vi "P116WriteAuto.vi"(8 "error in (no error)":errorcluster, 9 "NuevoRT":T1, 10 "NuevoSP":T1, 11 "Comunicaciones":T2={"Flujo_1"="ASRL6::INSTR", "Brk1"=FALSE, "Flujo_2"="ASRL6::INSTR", "Brk2"=FALSE, "Flujo_3"="ASRL6::INSTR", "Brk3"=FALSE, "Flujo_4"="ASRL6::INSTR", "Brk4"=FALSE, "Eurothe"="ASRL6::INSTR", "Eurot"=FALSE, "Balanza"="ASRL6::INSTR", "Bal"=FALSE, "eValPos"="ASRL6::INSTR", "eVal"=FALSE, "flowbus"="ASRL6::INSTR", "fb"=FALSE}) -> (0 "error out":errorcluster, 1 "NuevoRT2":T1, 2 "NuevoSP2":T1)   [LabVIEW 2013]
uses:
  4xP116.ctl
  Controles/P2018 Com Control.ctl
  Eurotherm_Hardware_Module Control.ctl
  P2022 TB INCAR GLOBALES.vi
panel:
  out "arrayRT":dbl[](array[numeric])
  out "arraySP":dbl[](array[numeric])
  out "PV":T1
  out "WorkingSP":T1
  out "TargetSP":T1
  in  "Cancel":bool
  in  "Write":bool
  out "Enable(T)":bool=TRUE
  out "VISA Promux":refnum<visa-resource-name>
  in  "Delay Time (s)":dbl=0.1
  # "Programando controladores P116"
  # "C"
  # "ARRIBA"
  # "C/min"
  # "C"
  # "ABAJO"
  # "C/min"
  # "C"
  # "CINTAS"
  # "C/min"
  # "C"
  # "LECTOR"
  # "C/min"
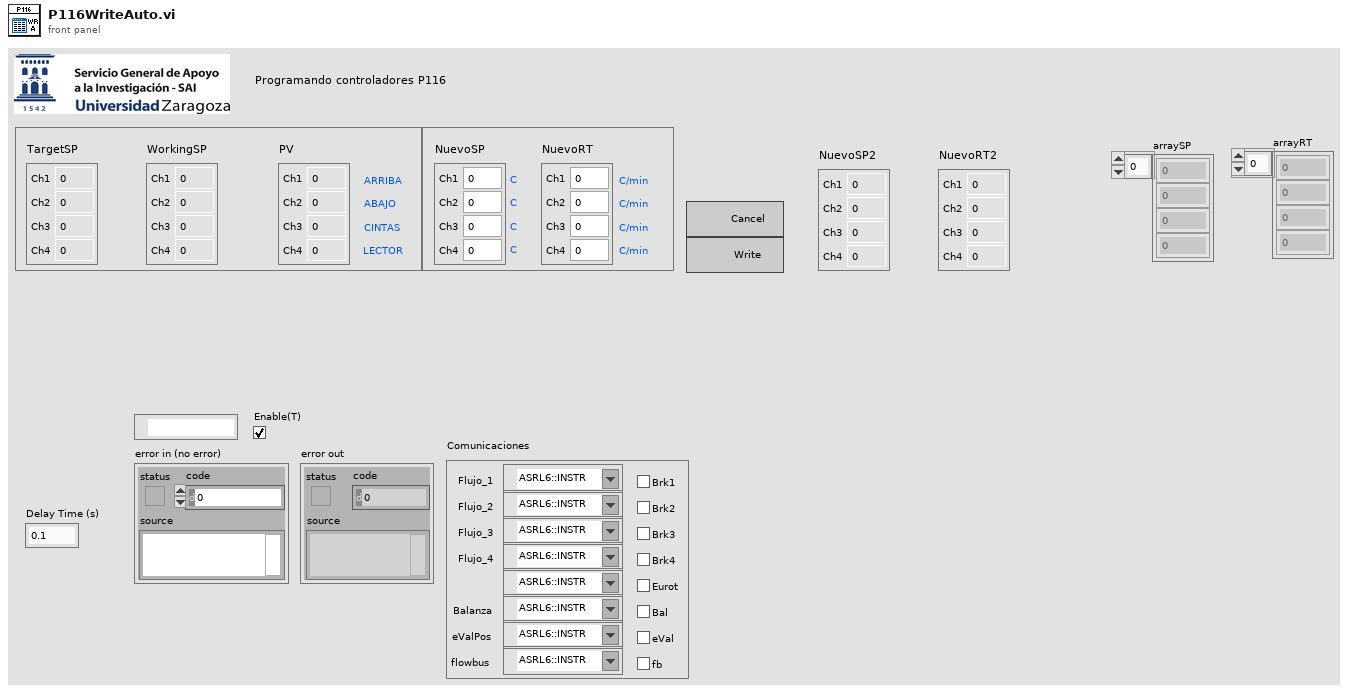
[diagram p1: front panel]
types:
  T1 = typedef "4xP116.ctl" = cluster{"Ch1":dbl, "Ch2":dbl, "Ch3":dbl, "Ch4":dbl}
  T2 = typedef "P2018 Com Control.ctl" = cluster{"Flujo_1":refnum<visa-resource-name>, "Brk1":bool, "Flujo_2":refnum<visa-resource-name>, "Brk2":bool, "Flujo_3":refnum<visa-resource-name>, "Brk3":bool, "Flujo_4":refnum<visa-resource-name>, "Brk4":bool, "Eurothe":refnum<visa-resource-name>, "Eurot":bool, "Balanza":refnum<visa-resource-name>, "Bal":bool, "eValPos":refnum<visa-resource-name>, "eVal":bool, "flowbus":refnum<visa-resource-name>, "fb":bool}
  T3 = typedef "P2018 Eurotherm Control.ctl" = cluster{"TargetSP":T1, "WorkingSP":T1, "Temperatura":T1, "Error":bool, "Date":string, "Delay(s)":dbl, "RateSP":T1, "Potencia":T1}
  T4 = typedef "Eurotherm_Hardware_Module Control.ctl" = enum16{"Initialize", "Write SP", "Read SP+PV", "Write Rate", "Set P", "Set I", "Set D", "Shutdown"}
  T5 = enum16{"Add 1", "Add 2", "Add 10", "Add 11", "Add 12", "Add 13"}[]
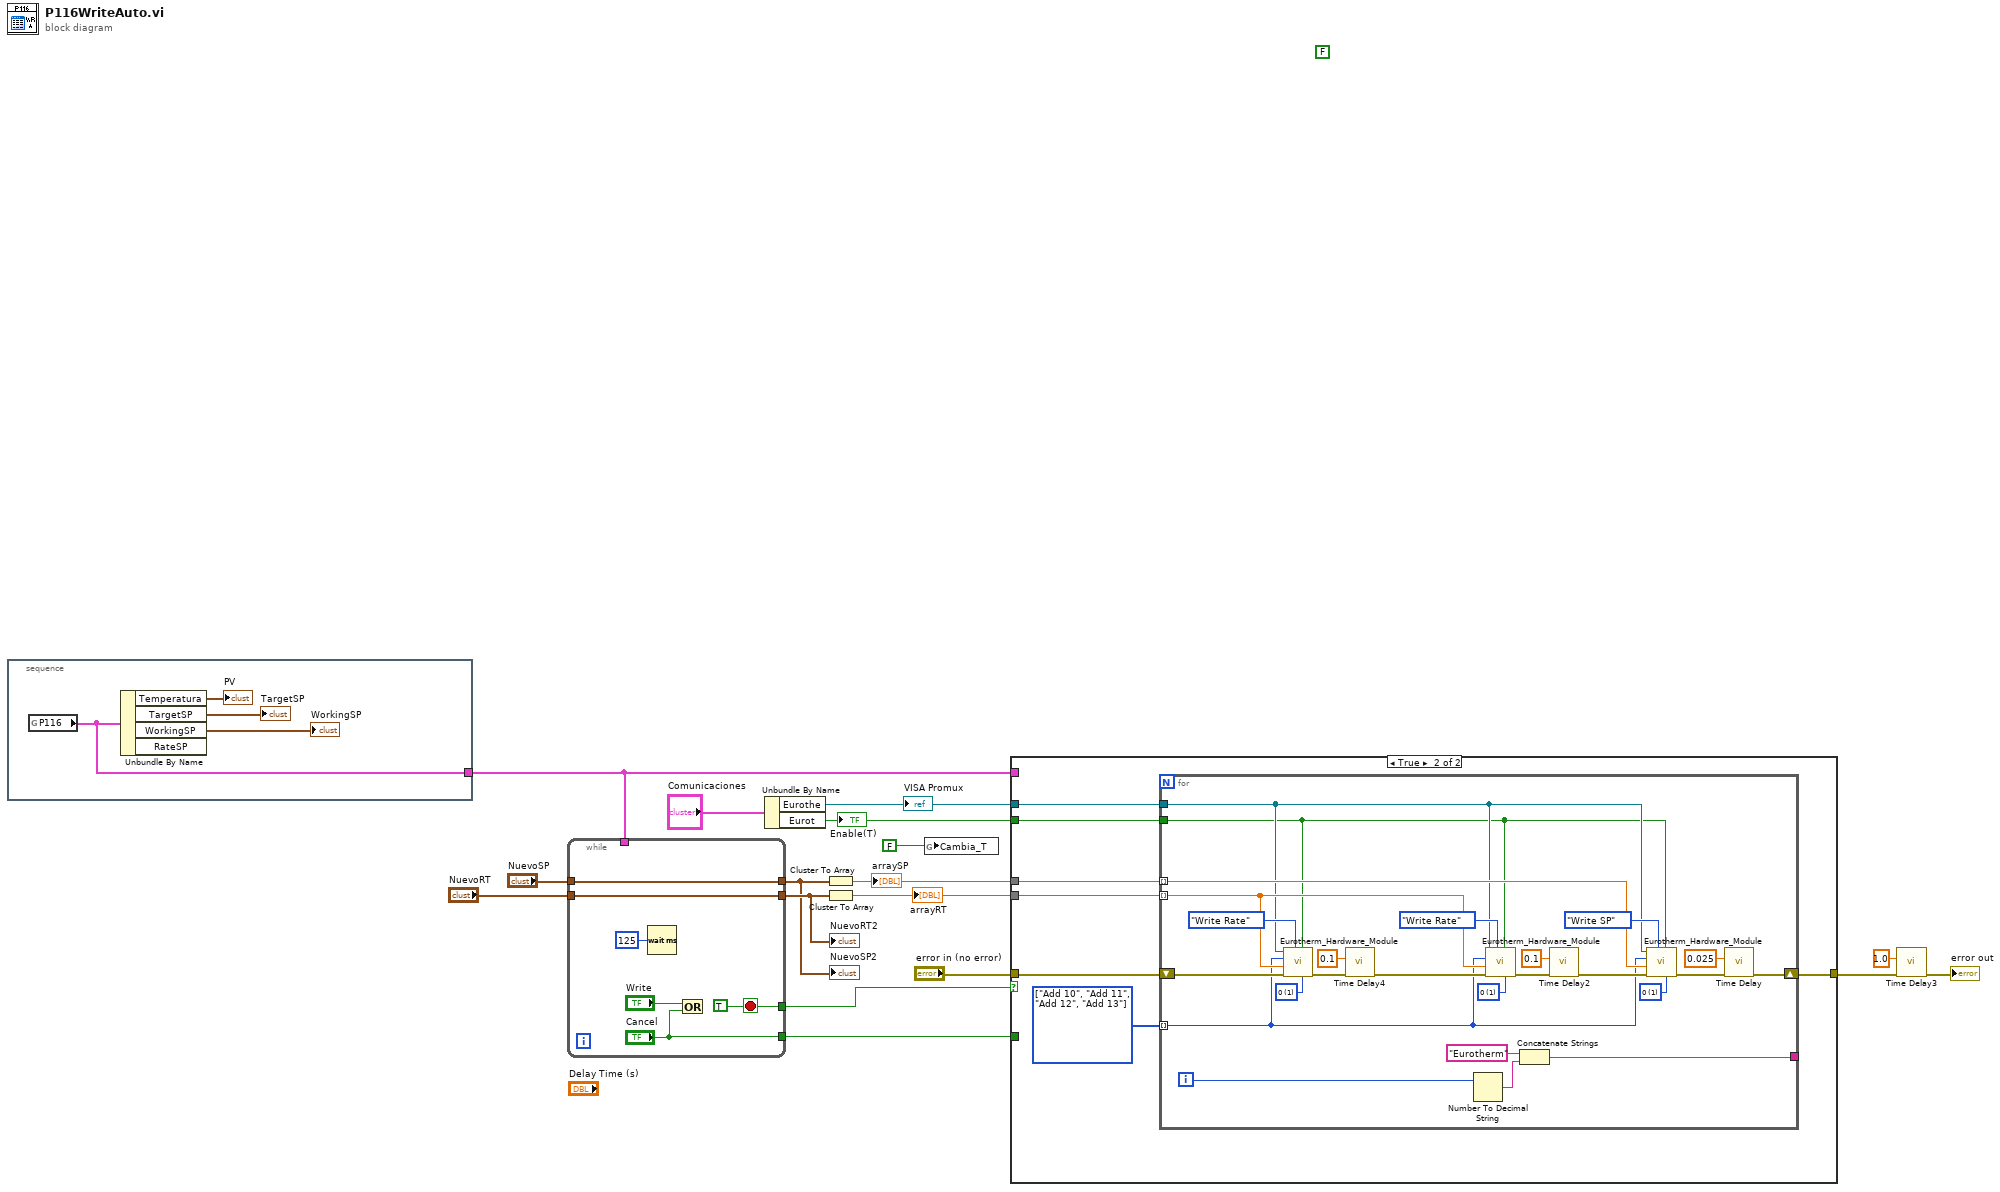
[diagram p0: block diagram]
diagram:
  (unwired) FALSE
  n1 = stacked-sequence {
    tunnel: [w18] -> w10
    frame #0 {
      n2 = global read "P2022 TB INCAR GLOBALES.vi" "P116"() -> (w18:T3)
      n3 = Unbundle By Name(w18) -> ("Temperatura"=→"PV":T1, "TargetSP"=→"TargetSP":T1, "WorkingSP"=→"WorkingSP":T1)  [unwired: 1 out]
    }
  }
  n4 = while {
    tunnel: ["Cancel"] -> w16
    tunnel: [w23] -> w8
    tunnel: [w24] -> w9
    tunnel: w10 -> [_]
    tunnel: "NuevoRT" -> [w24]
    tunnel: "NuevoSP" -> [w23]
    tunnel: [w22] -> w1
    stop <- w22 stop-if-true
    w22 = TRUE
    n5 = Wait (ms)(milliseconds to wait=u32 125) -> ()  [unwired: 1 out]
    n6 = Or(x="Write", y="Cancel") -> ()  [unwired: 1 out]
  }
  "NuevoSP2" <- w8
  "NuevoRT2" <- w9
  n7 = Unbundle By Name("Comunicaciones") -> ("Eurothe"=w11:refnum<visa-resource-name>, "Eurot"=w17:bool)
  "Enable(T)" <- w17
  "VISA Promux" <- w11
  n8 = Cluster To Array(cluster=w8) -> (array=w14:dbl[])
  "arraySP" <- w14
  n9 = Cluster To Array(cluster=w9) -> (array=w13:dbl[])
  "arrayRT" <- w13
  n10 = global write "P2022 TB INCAR GLOBALES.vi" "Cambia_T"(FALSE ("ChangeT")) -> ()
  n11 = case shown="True" w1 {
    tunnel: w17 -> [_ w34]
    tunnel: w16 -> [_ _]
    tunnel: "error in (no error)" -> [w28 w33]
    tunnel: w14 -> [_ w31]
    tunnel: w13 -> [_ w32]
    tunnel: w11 -> [_ w35]
    tunnel: w10 -> [_ _]
    tunnel: [w28 w29] -> w5
    frame False {
    }
    frame True {
      w30 = T5 [enum."Add 10", enum."Add 11", enum."Add 12", enum."Add 13"] items=["Add 1", "Add 2", "Add 10", "Add 11", "Add 12", "Add 13"]
      n12 = for {
        tunnel: w30 -> [w38] mode=indexing
        shift-right: [w51] -> w29
        shift-left: w33 -> [w55]
        tunnel: [w58] -> _
        tunnel: w31 -> [w53] mode=indexing
        tunnel: w32 -> [w39] mode=indexing
        tunnel: w35 -> [w37]
        tunnel: w34 -> [w36]
        i -> [w50]
        w40 = u16 1 items=["0"=1, "1"=10, "2"=100] ("Decimales")
        w49 = u16 1 items=["0"=1, "1"=10, "2"=100] ("Decimales")
        w48 = u16 1 items=["0"=1, "1"=10, "2"=100] ("Decimales")
        n13 = call "Eurotherm_Hardware_Module.vi"("Decimales"=w49, "Eurotherm (T:Enable)"=w36, "Command"=Eurotherm_Hardware_Module_Control."Write Rate", "error in (no error)"=w55, "Value"=w39, "Address"=w38, "VISA resource name"=w37) -> ("error out"=w42:errorcluster)  [unwired: 2 in, 2 out]
        n14 = call "Time Delay4"("error in (no error)"=w42, "Delay Time (s)"=0.1) -> ("error out"=w43:errorcluster)  [unwired: 9 in]
        n15 = Number To Decimal String(number=w50) -> (decimal integer string=w59:string)  [unwired: 1 in]
        n16 = call "Eurotherm_Hardware_Module.vi"("Decimales"=w40, "Eurotherm (T:Enable)"=w36, "Command"=Eurotherm_Hardware_Module_Control."Write Rate", "error in (no error)"=w43, "Value"=w39, "Address"=w38, "VISA resource name"=w37) -> ("error out"=w41:errorcluster)  [unwired: 2 in, 2 out]
        n17 = Concatenate Strings("Eurotherm" ("error source (\" \")"), w59) -> (w58:string)
        n18 = call "Time Delay2"("error in (no error)"=w41, "Delay Time (s)"=0.1) -> ("error out"=w46:errorcluster)  [unwired: 9 in]
        n19 = call "Eurotherm_Hardware_Module.vi"("Decimales"=w48, "Eurotherm (T:Enable)"=w36, "Command"=Eurotherm_Hardware_Module_Control."Write SP", "error in (no error)"=w46, "Value"=w53, "Address"=w38, "VISA resource name"=w37) -> ("error out"=w52:errorcluster)  [unwired: 2 in, 2 out]
        n20 = call "Time Delay"("error in (no error)"=w52, "Delay Time (s)"=0.025) -> ("error out"=w51:errorcluster)  [unwired: 9 in]
      }
    }
  }
  n21 = call "Time Delay3"("error in (no error)"=w5, "Delay Time (s)"=1.0) -> ("error out"=→"error out":errorcluster)  [unwired: 9 in]
